vi "Mapping.vi"(7 "VirtualMapping":u16[][](array[numeric]), 8 "error in (no error)":errorcluster, 9 "Queues":T3, 10 "Array Parsed Expression":T1[](array[typedef]), 11 "Variable Data In":T4) -> (0 "error out":errorcluster, 2 "Array Parsed Expression Out":T1[](array[typedef]), 3 "Variable Data Out":T4)   [LabVIEW 2014, in "MathLoop.lvlib"]
doc: "Mapea la entrada de valores correspondientes de la Queues con los valores seteados por el usuario."
uses:
  MathLoop.lvlib
  APIs/Data Queue/Acquisition Data 1 Sample Cluster.ctl
  TypeDefs/ParsedExpression.ctl
  TypeDefs/typeMed.ctl
  APIs/Data Queue/WINFAS 2 Data Queue.lvlib
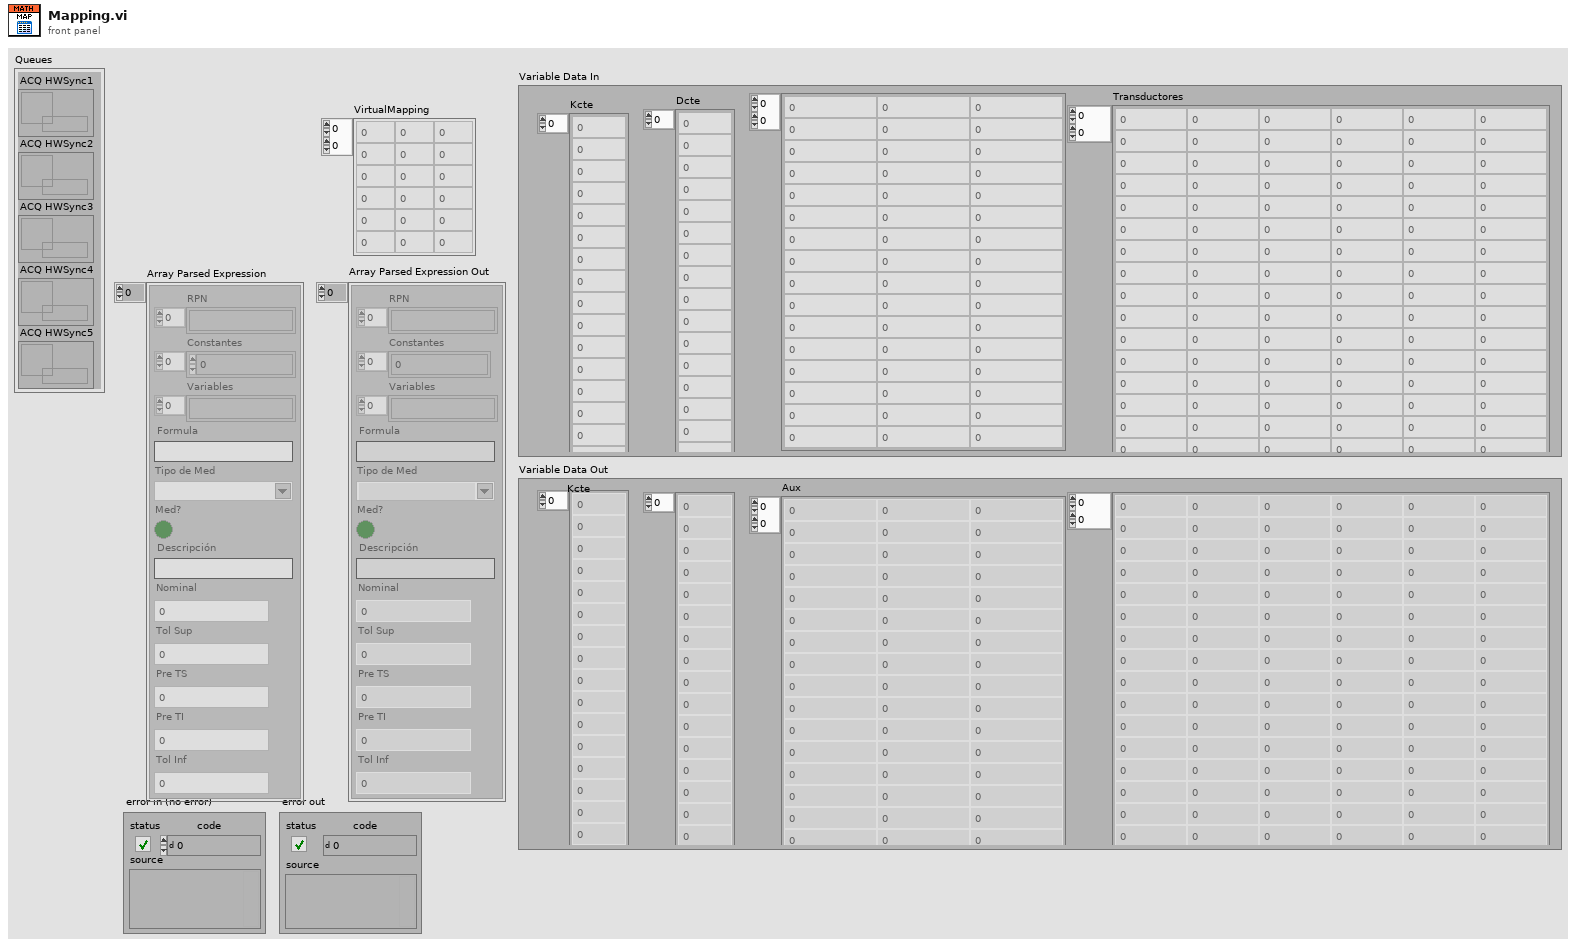
[diagram p1: front panel]
types:
  T1 = typedef "MathLoop.lvlib/ParsedExpression.ctl" = cluster{"RPN ":string[], "Constantes":sgl[], "Variables":string[], "Formula":string, "Tipo de Med":T2, "Med?":bool, "Descripción":string, "Nominal":sgl, "Tol Sup":sgl, "Pre TS":sgl, "Pre TI":sgl, "Tol Inf":sgl}
  T2 = typedef "MathLoop.lvlib/typeMed.ctl" = string
  T3 = cluster{"ACQ HWSync1":refnum<queue>, "ACQ HWSync2":refnum<queue>, "ACQ HWSync3":refnum<queue>, "ACQ HWSync4":refnum<queue>, "ACQ HWSync5":refnum<queue>}
  T4 = cluster{"Kcte":sgl[], "Dcte":sgl[], "Aux":sgl[][], "Transductores":sgl[][]}
  T5 = typedef "WINFAS 2 Data Queue.lvlib/Acquisition Data 1 Sample Cluster.ctl" = cluster{"TDX":sgl[], "Encoder":sgl}
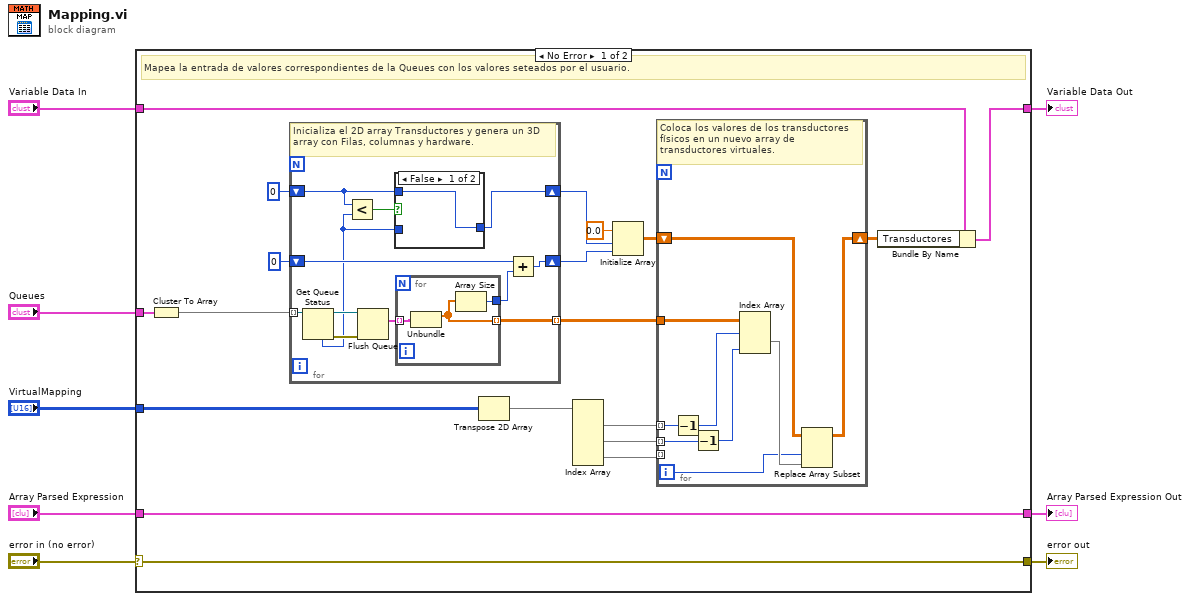
[diagram p0: block diagram]
diagram:
  n1 = case shown="No Error" "error in (no error)" {
    selector: "error in (no error)" -> [w17 w54]
    tunnel: [w21 w56] -> w8
    tunnel: "Variable Data In" -> [w20 w56]
    tunnel: "VirtualMapping" -> [w19 _]
    tunnel: [w18 w55] -> w2
    tunnel: "Array Parsed Expression" -> [w18 w55]
    tunnel: [w17 w54] -> w4
    tunnel: "Queues" -> [w16 _]
    frame No Error {
      # "Mapea la entrada de valores correspondientes de la Queues con los valores seteados por el usuario."
      n2 = Cluster To Array(cluster=w16) -> (array=w11:refnum<queue>[])
      n3 = for {
        tunnel: w11 -> [w37] mode=indexing
        tunnel: [w38] -> w23 mode=indexing
        shift-right: [w32] -> w13
        shift-left: 0 -> [w34]
        shift-right: [w29] -> w12
        shift-left: 0 -> [w28]
        # "Inicializa el 2D array Transductores y genera un 3D array con Filas, columnas y hardware."
        n4 = Get Queue Status(queue=w37) -> (queue out=w36:refnum<queue>, error out=w35:errorcluster, # elements in queue=w30:i32)  [unwired: 2 in, 5 out]
        n5 = Less?(x=w28, y=w30) -> (x < y?=w31:bool)
        n6 = Flush Queue(queue=w36, error in (no error)=w35) -> (remaining elements=w39:T5[])  [unwired: 2 out]
        n7 = case shown="False" w31 {
          tunnel: [w40 w41] -> w29
          tunnel: w30 -> [_ w41]
          tunnel: w28 -> [w40 _]
          frame False {
          }
          frame True {
          }
        }
        n8 = for {
          tunnel: w39 -> [w44] mode=indexing
          tunnel: [w43] -> w38 mode=indexing
          tunnel: [w42] -> w33
          n9 = Unbundle(w44) -> ("TDX"=w43:sgl[])  [unwired: 1 out]
          n10 = Array Size(array=w43) -> (size(s)=w42:i32)
        }
        n11 = Add(x=w34, y=w33) -> (x+y=w32:i32)
      }
      n12 = Transpose 2D Array(2D array=w19) -> (transposed array=w24:u16[][])
      n13 = Index Array(array=w24) -> (element #1=w25:u16[], element #2=w27:u16[], element #3=w26:u16[])  [unwired: 6 in]
      n14 = Initialize Array(sgl 0.0 ("element"), w12, w13) -> (w15:sgl[][])
      n15 = for {
        tunnel: w25 -> [w49] mode=indexing
        tunnel: w27 -> [w47] mode=indexing
        tunnel: w26 -> [_] mode=indexing
        shift-right: [w52] -> w22
        shift-left: w15 -> [w53]
        tunnel: w23 -> [w51]
        i -> [w45]
        # "Coloca los valores de los transductores físicos en un nuevo array de transductores virtuales."
        n16 = Decrement(x=w49) -> (x-1=w48:u16)
        n17 = Decrement(x=w47) -> (x-1=w46:u16)
        n18 = Index Array(array=w51, index (dim 0)=w48, index (dim 2)=w46) -> (element=w50:sgl[])  [unwired: 1 in]
        n19 = Replace Array Subset(array=w53, new element=w50, index (col)=w45) -> (w52:sgl[][])  [unwired: 1 in]
      }
      n20 = Bundle By Name(cluster=w20, "Transductores"=w22) -> (w21:T4)
    }
    frame Error {
    }
  }
  "error out" <- w4
  "Variable Data Out" <- w8
  "Array Parsed Expression Out" <- w2
